vi "UPDATE RING LISTS.vi"(11 "SEARCH DATABASE REFERENCES":T1) -> ()   [LabVIEW 2019]
uses:
  Controls/Custom Calendar/Custom Calendar.xctl
  <vilib>/Utility/miscctls.llb/LVStringsAndValuesArrayTypeDef_U16.ctl
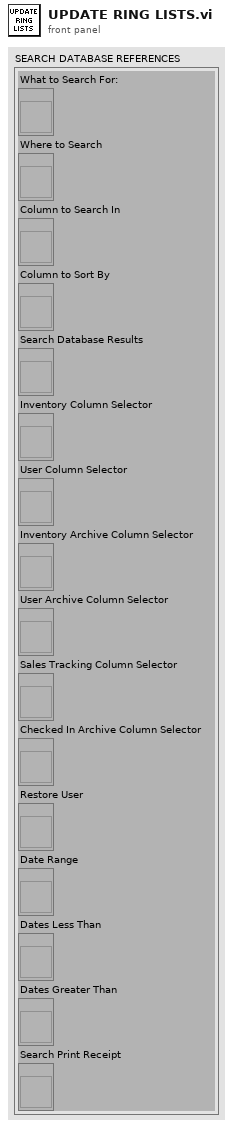
[diagram p1: front panel]
types:
  T1 = cluster{"What to Search For:":refnum<vi>, "Where to Search":refnum<vi>, "Column to Search In":refnum<vi>, "Column to Sort By":refnum<vi>, "Search Database Results":refnum<vi>, "Inventory Column Selector":refnum<vi>, "User Column Selector":refnum<vi>, "Inventory Archive Column Selector":refnum<vi>, "User Archive Column Selector":refnum<vi>, "Sales Tracking Column Selector":refnum<vi>, "Checked In Archive Column Selector":refnum<vi>, "Restore User":refnum<vi>, "Date Range":refnum<vi>, "Dates Less Than":refnum<vi>, "Dates Greater Than":refnum<vi>, "Search Print Receipt":refnum<vi>}
  T2 = typedef "LVStringsAndValuesArrayTypeDef_U16.ctl" = cluster{"String":string, "Value":u16}[]
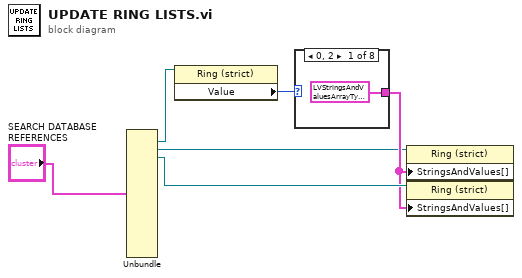
[diagram p0: block diagram]
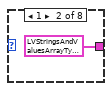
[diagram p2: hidden frame]
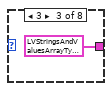
[diagram p3: hidden frame]
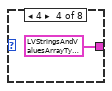
[diagram p4: hidden frame]
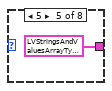
[diagram p5: hidden frame]
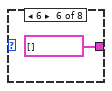
[diagram p6: hidden frame]
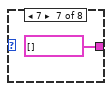
[diagram p7: hidden frame]
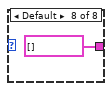
[diagram p8: hidden frame]
diagram:
  n1 = Unbundle("SEARCH DATABASE REFERENCES") -> ("Where to Search"=w6:refnum<vi>, "Column to Search In"=w2:refnum<vi>, "Column to Sort By"=w4:refnum<vi>)  [unwired: 13 out]
  n2 = property class="Ring (strict)"(reference=w6) -> ("Value"=w5:u16)  [unwired: 1 in, 2 out]
  n3 = case shown="0, 2" w5 {
    tunnel: [T2 [{"String"="Identifier", "Value"=0}, {"String"="BYU ICN #", "Value"=1}, {"String"="Item Description", "Value"=2}, {"String"="Comments", "Value"=3}, {"String"="Checked Out Date", "Value"=4}, {"String"="Due Date", "Value"=5}, {"String"="Check Out Location", "Value"=6}, {"String"="Reminder Count", "Value"=7}, {"String"="Most Recent Reminder Date", "Value"=8}, {"String"="BYU ID #", "Value"=9}, {"String"="Building/Room", "Value"=10}, {"String"="Location in Room", "Value"=11}, {"String"="Manual", "Value"=12}, {"String"="Manufacturer", "Value"=13}, {"String"="Model #", "Value"=14}, {"String"="Serial #", "Value"=15}, {"String"="Date Acquired", "Value"=16}] ("Strings And Values []") T2 [{"String"="BYU ID #", "Value"=0}, {"String"="First Name", "Value"=1}, {"String"="Last Name", "Value"=2}, {"String"="Phone Number", "Value"=3}, {"String"="Email", "Value"=4}, {"String"="Department", "Value"=5}, {"String"="Graduation Status", "Value"=6}, {"String"="Anticipated Graduation Year", "Value"=7}, {"String"="Credit Score", "Value"=8}, {"String"="Date Added", "Value"=9}, {"String"="Graduation Clearance Date", "Value"=10}, {"String"="Picture File Name", "Value"=11}] ("Strings And Values []") T2 [{"String"="Date Disposed", "Value"=0}, {"String"="Disposal Method", "Value"=1}, {"String"="Auction #", "Value"=2}, {"String"="Date Inventory Office Emailed", "Value"=3}, {"String"="Disposal Notes", "Value"=4}, {"String"="Identifier", "Value"=5}, {"String"="BYU ICN #", "Value"=6}, {"String"="Item Description", "Value"=7}, {"String"="Comments", "Value"=8}, {"String"="Building/Room", "Value"=9}, {"String"="Location in Room", "Value"=10}, {"String"="Manual", "Value"=11}, {"String"="Manufacturer", "Value"=12}, {"String"="Model #", "Value"=13}, {"String"="Serial #", "Value"=14}, {"String"="Date Acquired", "Value"=15}] ("Strings And Values []") T2 [{"String"="BYU ID #", "Value"=0}, {"String"="First Name", "Value"=1}, {"String"="Last Name", "Value"=2}, {"String"="Phone Number", "Value"=3}, {"String"="Email", "Value"=4}, {"String"="Department", "Value"=5}, {"String"="Graduation Status", "Value"=6}, {"String"="Anticipated Graduation Year", "Value"=7}, {"String"="Credit Score", "Value"=8}, {"String"="Date Added", "Value"=9}, {"String"="Graduation Clearance Date", "Value"=10}, {"String"="Picture File Name", "Value"=11}, {"String"="Date Archived", "Value"=12}] ("Strings And Values []") T2 [{"String"="Identifier", "Value"=0}, {"String"="BYU ICN #", "Value"=1}, {"String"="Item Description", "Value"=2}, {"String"="Comments", "Value"=3}, {"String"="Checked Out Date", "Value"=4}, {"String"="Due Date", "Value"=5}, {"String"="Check Out Location", "Value"=6}, {"String"="Reminder Count", "Value"=7}, {"String"="Most Recent Reminder Date", "Value"=8}, {"String"="BYU ID #", "Value"=9}, {"String"="Building/Room", "Value"=10}, {"String"="Location in Room", "Value"=11}, {"String"="Manual", "Value"=12}, {"String"="Manufacturer", "Value"=13}, {"String"="Model #", "Value"=14}, {"String"="Serial #", "Value"=15}, {"String"="Date Acquired", "Value"=16}, {"String"="Date Checked In", "Value"=17}] ("Strings And Values []") T2 [] ("Strings And Values []") T2 [] ("Strings And Values []") T2 [] ("Strings And Values []")] -> w3
    frame 0, 2 {
    }
    frame 1 {
    }
    frame 3 {
    }
    frame 4 {
    }
    frame 5 {
    }
    frame 6 {
    }
    frame 7 {
    }
    frame Default {
    }
  }
  n4 = property class="Ring (strict)"(reference=w2, "StringsAndValues[]"=w3) -> ()  [unwired: 1 in, 2 out]
  n5 = property class="Ring (strict)"(reference=w4, "StringsAndValues[]"=w3) -> ()  [unwired: 1 in, 2 out]
